vi "RT Main v1.05.vi"() -> ()   [LabVIEW 2017]
doc: "Changelog:\n\nv0.9:\n- Autocycle"
uses:
  Controls/Auto Delays.ctl
  support/Controls/General Para.ctl
  support/Controls/All Inputs.ctl
  support/Controls/Index Details.ctl
  support/Controls/Auto Stats.ctl
  Controls/Auto Times.ctl
  Global Variables/RT GV.vi
  support/Message Queue/Enqueue Message (Single).vi
  Global Variables/FPGA GV.vi
  <vilib>/Utility/error.llb/Error Cluster From Error Code.vi
  <vilib>/rvi/errors/niLvFpgaAdjustHostInterfaceError.vi
  Global Variables/Network Globals.vi
  <vilib>/FPGAPlugInAG/Dynamic/niLvFpga_Close_Dynamic.vi
  <vilib>/rvi/interface/nirviReadWriteControl/nirviReadWriteControl.xnode
  Controls/FPGA Ref.ctl
  <vilib>/rvi/interface/nirviCloseFPGA/nirviCloseFPGA.xnode
  support/Message Queue/Message Queue.lvlib
  NiFpgaLv.dll
  <vilib>/rvi/interface/Simulation/niFpgaSimulationCallBeginRW.vi
panel:
  in  "Auto Para":T1={"Agitator Delays"=[250, 350], "TF Delays"=[700, 800, 2], "Insertion Delays"=[100, 500], "Cutting Delays"=[300, 300, 100], "PF Delays"=[250, 30000], "Measur. Delays"=[500.0, 188.9, 1.0], "Reject Delays"=[500], "BF Delays"=[1000, 1000]}
  in  "Stop Button 4":bool
  out "error out":errorcluster
  out "Wrong Message":string
  in  "Stop Button":bool
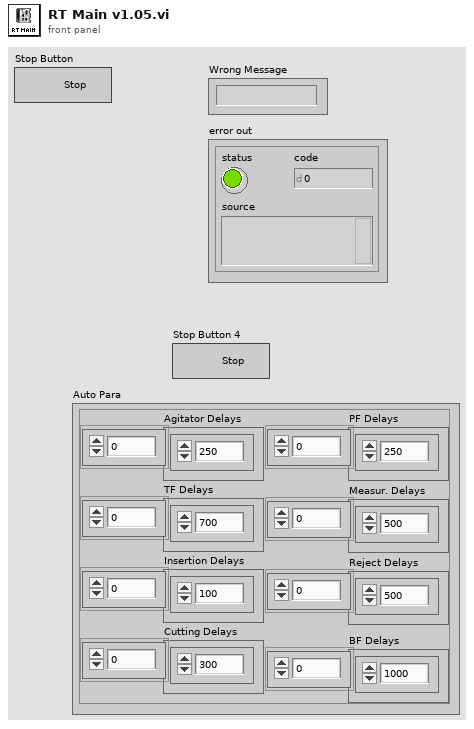
[diagram p1: front panel]
types:
  T1 = typedef "Auto Delays.ctl" = cluster{"Agitator Delays":u32[], "TF Delays":u32[], "Insertion Delays":u32[], "Cutting Delays":u32[], "PF Delays":u32[], "Measur. Delays":dbl[], "Reject Delays":u32[], "BF Delays":u32[]}
  T2 = typedef "FPGA Ref.ctl" = refnum<k20>
  T3 = cluster{"TL_Red":bool, "TL_Orange":bool, "TL_Green":bool, "TL_Buzzer":bool, "SOL_Index_Rotary_CW":bool, "SOL_Index_CNVR_Rotary_CCW":bool, "SOL_Index_CNVR_Stopper_Rear":bool, "SOL_Index_CNVR_Output _Separator _Rear":bool, "Bowl  Feeder_ ON":bool, "Pump_CNVR_Motor _ON":bool, "SOL_Gating_CYL_Rear":bool, "SOL_Tube_Feed_Agitatator":bool, "SOL_Tube_Feed_Gating_CYL":bool, "SOL_Insertion _CYL":bool, "SOL_Insertion_Clamp_CYL":bool, "SOL_Cutting_CYL":bool, "SOL_Cutting_Clamp_CYL":bool, "SOL_Insertion_Air_Nozzle":bool, "SOL_Measurement_CYL":bool, "SOL_Measure_Clamp_CYL":bool, "SOL_Rejection CYL_1":bool, "SOL_Rejection CYL_2":bool, "SOL_Rejection CYL_3":bool, "SOL_Rejection CYL_4":bool, "DO1.24":bool, "DO1.25":bool, "DO1.26":bool, "DO1.27":bool, "DO1.28":bool, "DO1.29":bool, "DO1.30":bool, "DO1.31":bool}
  T4 = typedef "General Para.ctl" = cluster{"Max. Cons.":dbl, "Offset 1":dbl, "Offset 2":dbl, "Offset 3":dbl, "Offset 4":dbl}
  T5 = typedef "All Inputs.ctl" = cluster{"DI 1":cluster{"Machine_ON":bool, "E_stop ":bool, "SW_Pressure":bool, "SW_Start ":bool, "SW_Reset":bool, "SW_Stop":bool, "SW_Door":bool, "RS_Index_Rotary_CW":bool, "RS_Index_Rotary_CCW":bool, "RS_Index_Stopper _Rear":bool, "RS_Index_Output_Separator_Rear":bool, "PES_Index_Pallet_Sensor":bool, "PES_Index_Output_Part Sensor":bool, "ICS_BF_Low_Level_1":bool, "ICS_BF_Low_Level_2":bool, "ICS_BF_Pump_CNVR_Full_1":bool, "ICS_BF_Pump_CNVR_Full_2":bool, "ICS_BF_Pump_CNVR_Full_3":bool, "ICS_BF_Pump_CNVR_Full_4":bool, "PES_PC_Pump Presence_1":bool, "PES_PC_Pump Presence_2":bool, "PES_PC_Pump Presence_3":bool, "PES_PC_Pump Presence_4":bool, "RS_PC_Gating_Front":bool, "PES_Pump_Interference":bool, "PES_TF_Low_Level":bool, "PES_Tube Presence_1":bool, "PES_Tube Presence_2":bool, "PES_Tube Presence_3":bool, "PES_Tube Presence_4":bool, "DI1.30":bool, "DI1.31":bool}, "DI 2":cluster{"RS_Agitatator_1_Rear ":bool, "RS_Agitatator_2_Rear ":bool, "RS_TF_Gating CYL_Rear":bool, "RS_Insertion_1_Rear":bool, "RS_Insertion_1_Front":bool, "RS_Insertion _2_Rear":bool, "RS_Insertion _2_Front":bool, "RS_Insertion _3_Rear":bool, "RS_Insertion _3_Front":bool, "RS_Insertion _4_Rear":bool, "RS_Insertion _4_Front":bool, "RS_Insertion_Clamp_Rear":bool, "RS_Cutting_Rear":bool, "RS_Cutting_Clamp _Rear":bool, "RS_Measurement_1_Rear":bool, "RS_Measurement_2_Rear":bool, "RS_Measurement_3_Rear":bool, "RS_Measurement_4_Rear":bool, "RS_Measure_Clamp_Rear":bool, "RS_Rejection_1_Rear":bool, "RS_Rejection_2_Rear":bool, "RS_Rejection_3_Rear":bool, "RS_Rejection_4_Rear":bool, "DI2.23":bool, "DI2.24":bool, "DI2.25":bool, "DI2.26":bool, "DI2.27":bool, "DI2.28":bool, "DI2.29":bool, "DI2.30":bool, "DI2.31":bool}, "IAS 1":dbl, "IAS 2":dbl, "IAS 3":dbl, "IAS 4":dbl, "DO 1":cluster{"TL_Red":bool, "TL_Orange":bool, "TL_Green":bool, "TL_Buzzer":bool, "SOL_Index_Rotary_CW":bool, "SOL_Index_CNVR_Rotary_CCW":bool, "SOL_Index_CNVR_Stopper_Rear":bool, "SOL_Index_CNVR_Output _Separator _Rear":bool, "Bowl  Feeder_ ON 1":bool, "Pump_CNVR_Motor _ON":bool, "SOL_PC_Gating_CYL_Rear":bool, "SOL_Tube_Feed_Agitatator":bool, "SOL_Tube_Feed_Gating_CYL":bool, "SOL_Insertion _CYL":bool, "SOL_Insertion_Clamp_CYL":bool, "SOL_Cutting_CYL":bool, "SOL_Cutting_Clamp_CYL":bool, "SOL_Insertion_Air_Nozzle":bool, "SOL_Measurement_CYL":bool, "DO1.19":bool, "SOL_Rejection CYL_1":bool, "SOL_Rejection CYL_2":bool, "SOL_Rejection CYL_3":bool, "SOL_Rejection CYL_4":bool, "Bowl  Feeder_ ON 2":bool, "SOL_BF_BlowerON":bool, "SOL_BF1_Track1":bool, "SOL_BF1_Track2":bool, "SOL_BF2_Track1":bool, "SOL_BF2_Track2":bool, "DO1.30":bool, "DO1.31":bool}}
  T6 = typedef "Index Details.ctl" = cluster{"Time (ms)":u32, "Waveform Graph":i16[]}
  T7 = cluster{T1, "Reject Pallets":cluster{"Reject 1":bool, "Reject 2":bool, "Reject 3":bool, "Reject 4":bool}}
  T8 = typedef "Auto Stats.ctl" = cluster{"Time-Stamp":timestamp, "Auto Times":T9, "Measurements":cluster{"1":dbl, "2":dbl, "3":dbl, "4":dbl}, "Outputs":cluster{"Good Parts":u32, "Reject Parts":u32}, "Cycle Time":dbl, "Remarks":string}
  T9 = typedef "Auto Times.ctl" = cluster{"Index Time":u32, "TF Time":u32, "Insertion Time":u32, "Cutting Time":u32, "PF Time":u32, "Meas. Time":u32, "Reject Time":u32}
  T10 = cluster{string, dbl, "cluster":cluster{"Auto Para":T1, "General Para":T4}}
  T11 = cluster{"TL_Red":bool, "TL_Orange":bool, "TL_Green":bool, "TL_Buzzer":bool, "SOL_Index_Rotary_CW":bool, "SOL_Index_CNVR_Rotary_CCW":bool, "SOL_Index_CNVR_Stopper_Rear":bool, "SOL_Index_CNVR_Output _Separator _Rear":bool, "Bowl Feeder_ ON1":bool, "Pump_CNVR_Motor _ON":bool, "SOL_PC_Gating_CYL_Rear":bool, "SOL_Tube_Feed_Agitatator":bool, "SOL_Tube_Feed_Gating_CYL":bool, "SOL_Insertion _CYL":bool, "SOL_Insertion_Clamp_CYL":bool, "SOL_Cutting_CYL":bool, "SOL_Cutting_Clamp_CYL":bool, "SOL_Insertion_Air_Nozzle":bool, "SOL_Measurement_CYL":bool, "DO1.19":bool, "SOL_Rejection CYL_1":bool, "SOL_Rejection CYL_2":bool, "SOL_Rejection CYL_3":bool, "SOL_Rejection CYL_4":bool, "Bowl Feeder_ON2":bool, "SOL_BF_BlowerON":bool, "SOL_BF1_Track1":bool, "SOL_BF1_Track2":bool, "SOL_BF2_Track1":bool, "SOL_BF2_Track2":bool, "DO1.30":bool, "DO1.31":bool}
  T12 = cluster{"Machine_ON":bool, "E_stop ":bool, "SW_Pressure":bool, "SW_Start ":bool, "SW_Reset":bool, "SW_Stop":bool, "SW_Door":bool, "RS_Index_Rotary_CW":bool, "RS_Index_Rotary_CCW":bool, "RS_Index_Stopper _Rear":bool, "RS_Index_Output_Separator_Rear":bool, "PES_Index_Pallet_Sensor":bool, "PES_Index_Output_Part Sensor":bool, "ICS_BF_Low_Level_1":bool, "ICS_BF_Low_Level_2":bool, "ICS_BF_Pump_CNVR_Full_1":bool, "ICS_BF_Pump_CNVR_Full_2":bool, "ICS_BF_Pump_CNVR_Full_3":bool, "ICS_BF_Pump_CNVR_Full_4":bool, "PES_PC_Pump Presence_1":bool, "PES_PC_Pump Presence_2":bool, "PES_PC_Pump Presence_3":bool, "PES_PC_Pump Presence_4":bool, "RS_PC_Gating_Front":bool, "PES_Pump_Interference":bool, "PES_TF_Low_Level":bool, "PES_Tube Presence_1":bool, "PES_Tube Presence_2":bool, "PES_Tube Presence_3":bool, "PES_Tube Presence_4":bool, "DI1.30":bool, "DI1.31":bool}
  T13 = cluster{"RS_Agitatator_1_Rear ":bool, "RS_Agitatator_2_Rear ":bool, "RS_TF_Gating CYL_Rear":bool, "RS_Insertion_1_Rear":bool, "RS_Insertion_1_Front":bool, "RS_Insertion _2_Rear":bool, "RS_Insertion _2_Front":bool, "RS_Insertion _3_Rear":bool, "RS_Insertion _3_Front":bool, "RS_Insertion _4_Rear":bool, "RS_Insertion _4_Front":bool, "RS_Insertion_Clamp_Rear":bool, "RS_Cutting_Rear":bool, "RS_Cutting_Clamp _Rear":bool, "RS_Measurement_1_Rear":bool, "RS_Measurement_2_Rear":bool, "RS_Measurement_3_Rear":bool, "RS_Measurement_4_Rear":bool, "DI2.18":bool, "RS_Rejection_1_Rear":bool, "RS_Rejection_2_Rear":bool, "RS_Rejection_3_Rear":bool, "RS_Rejection_4_Rear":bool, "DI2.23":bool, "DI2.24":bool, "DI2.25":bool, "DI2.26":bool, "DI2.27":bool, "DI2.28":bool, "DI2.29":bool, "DI2.30":bool, "DI2.31":bool}
  T14 = cluster{"Array":string[][], "Machine Status":string}
  T15 = cluster{"Measurements":cluster{"1":dbl, "2":dbl, "3":dbl, "4":dbl}, "Reject Pallets":cluster{"Reject 1":bool, "Reject 2":bool, "Reject 3":bool, "Reject 4":bool}}
  T16 = cluster{"Auto Times":T9, "Results":cluster{"Measurements":cluster{"1":dbl, "2":dbl, "3":dbl, "4":dbl}, "Reject Pallets":cluster{"Reject 1":bool, "Reject 2":bool, "Reject 3":bool, "Reject 4":bool}}, "OutputCount":u32, "error out":errorcluster}
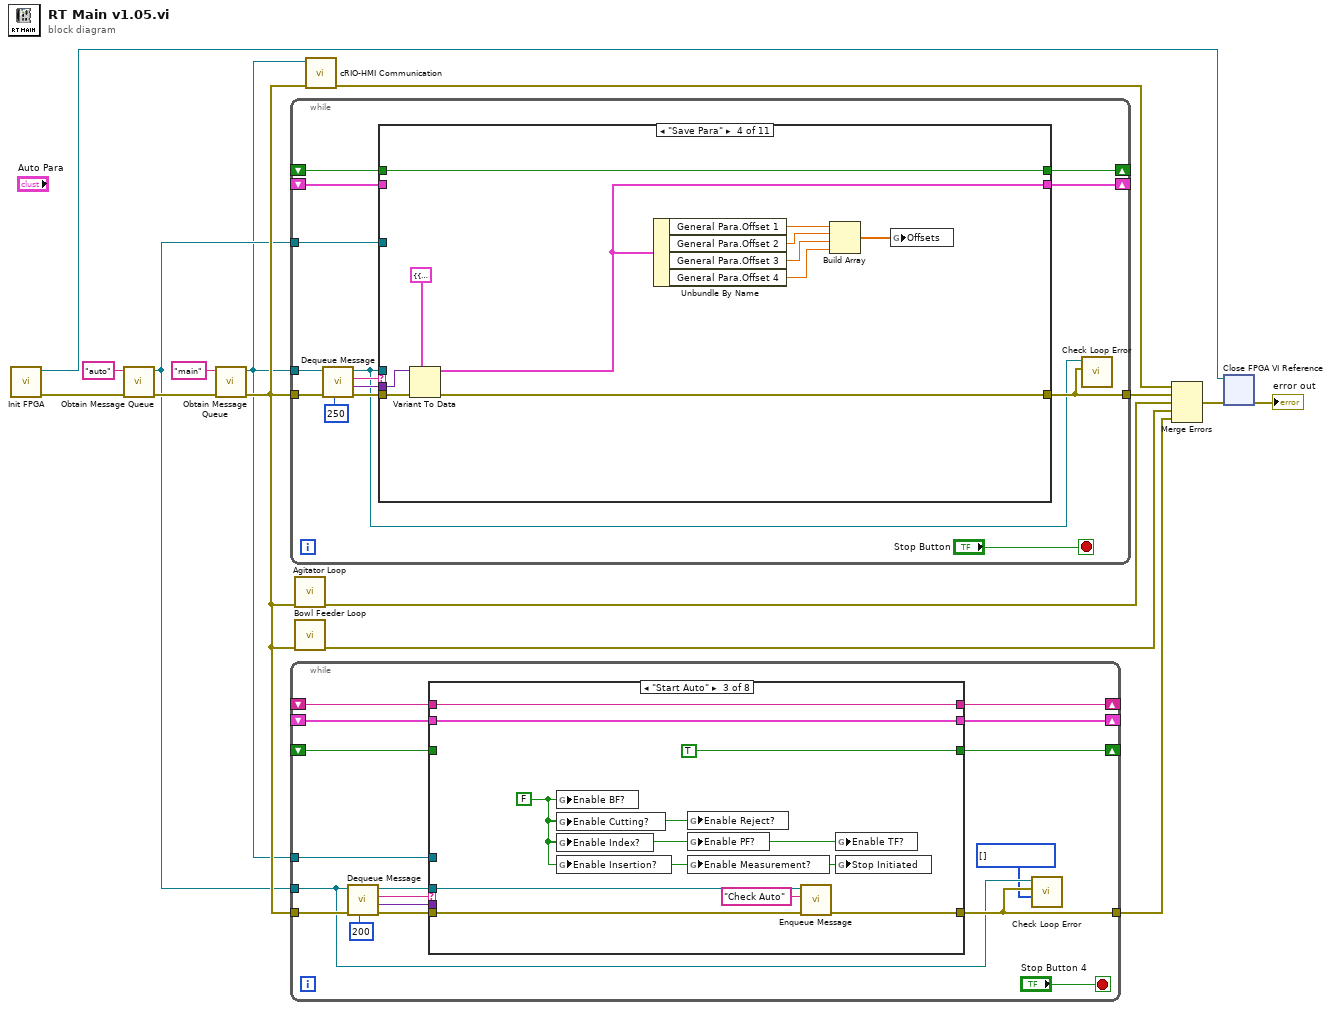
[diagram p0: block diagram]
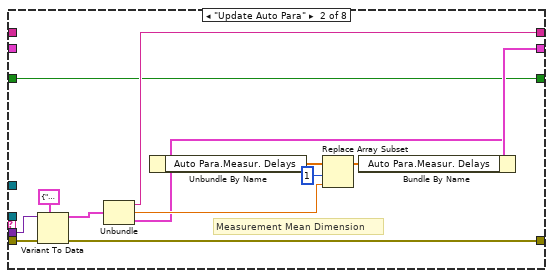
[diagram p3: hidden frame]
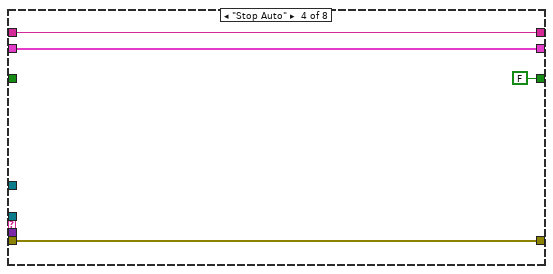
[diagram p4: hidden frame]
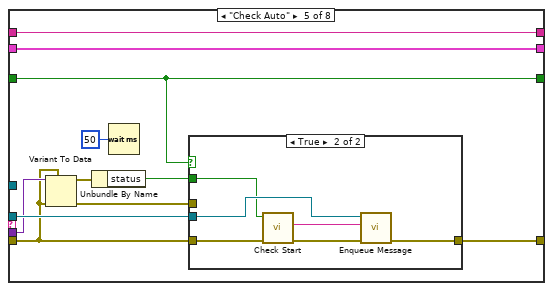
[diagram p5: hidden frame]
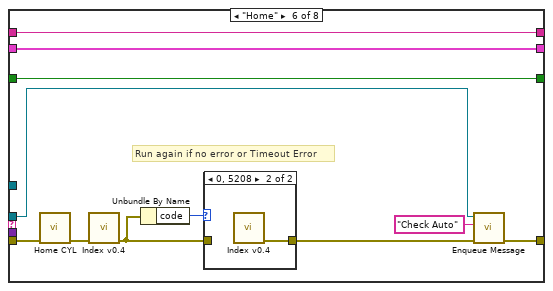
[diagram p7: hidden frame]
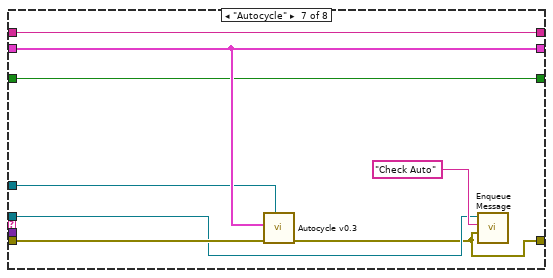
[diagram p9: hidden frame]
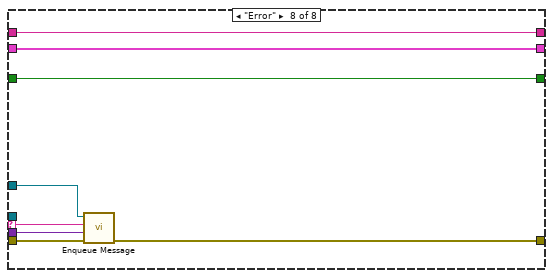
[diagram p10: hidden frame]
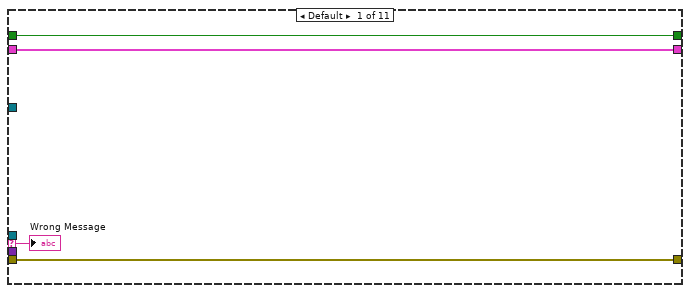
[diagram p11: hidden frame]
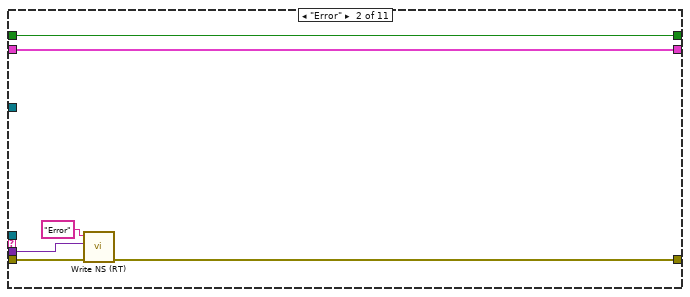
[diagram p12: hidden frame]
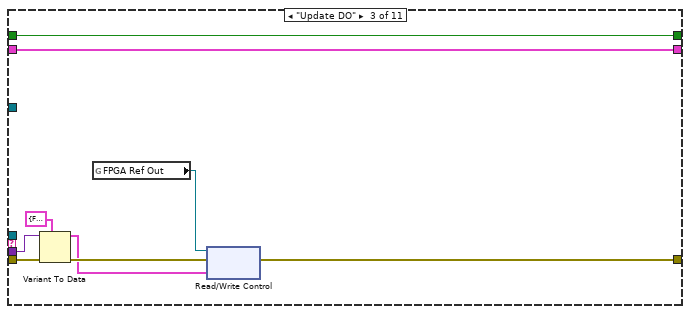
[diagram p13: hidden frame]
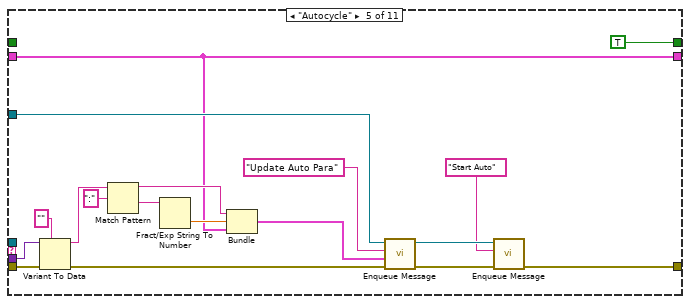
[diagram p14: hidden frame]
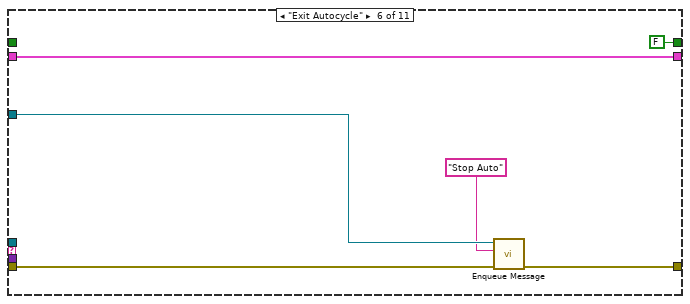
[diagram p15: hidden frame]
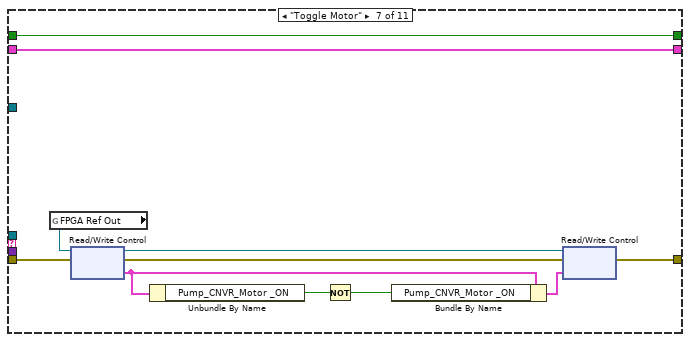
[diagram p16: hidden frame]
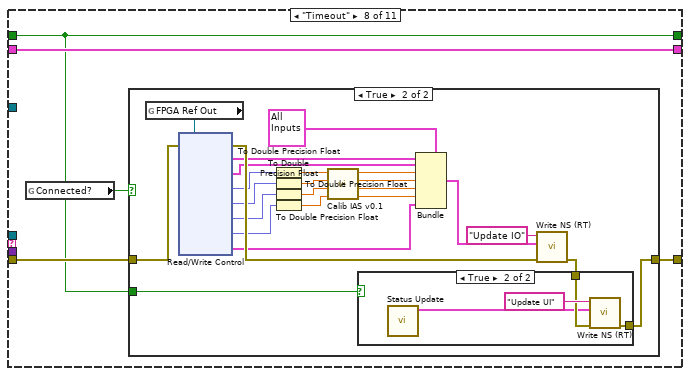
[diagram p17: hidden frame]
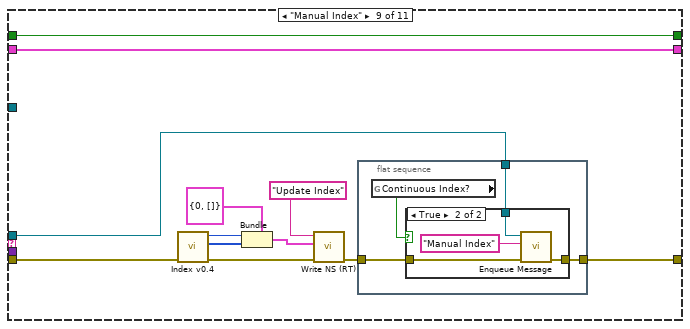
[diagram p20: hidden frame]
diagram:
  n1 = call "Init FPGA.vi"() -> ("error out"=w4:errorcluster, "FPGA Ref Out"=w9:T2)  [unwired: 10 in]
  n2 = call "Obtain Message Queue.vi"("error in (no error)"=w4, "name"="auto") -> ("error out"=w3:errorcluster, "Message Queue"=w2:refnum<queue>)  [unwired: 8 in]
  n3 = call "Obtain Message Queue.vi"("error in (no error)"=w3, "name"="main") -> ("error out"=w8:errorcluster, "Message Queue"=w1:refnum<queue>)  [unwired: 8 in]
  n4 = while {
    tunnel: w8 -> [w28]
    tunnel: w1 -> [w27]
    tunnel: [w23] -> w15
    tunnel: w2 -> [w20]
    shift-right: [w18] -> _
    shift-left: _ -> [w19]
    shift-right: [w16] -> _
    shift-left: _ -> [w17]
    stop <- "Stop Button" stop-if-true
    n5 = call "Dequeue Message.vi"("timeout"=250, "error in (no error)"=w28, "Message Queue"=w27) -> ("error out"=w26:errorcluster, "Message Data"=w24:variant, "Message"=w25:string, "dup Message Queue"=w22:refnum<queue>)  [unwired: 5 in]
    n6 = case shown="\"Save Para\"" w25 {
      selector: w25 -> [w33 _ _ _ _ _ _ _ _ _ _]
      tunnel: w26 -> [w32 w38 w48 w59 w77 w83 w93 w98 w141 w168 w178]
      tunnel: w22 -> [_ _ _ _ _ _ _ _ w133 _ _]
      tunnel: w24 -> [_ w36 w47 w58 w76 _ _ _ _ w167 w177]
      tunnel: [w32 w37 w43 w57 w63 w80 w91 w99 w134 w163 w174] -> w23
      tunnel: w20 -> [_ _ _ _ w69 w82 _ _ _ _ _]
      tunnel: w19 -> [w31 w39 w41 _ w66 w81 w85 w96 w131 w154 w173]
      tunnel: [w31 w39 w41 w54 w66 w81 w85 w96 w131 w154 w173] -> w18
      tunnel: w17 -> [w30 w34 w40 w56 _ _ w84 w95 w130 w151 w169]
      tunnel: [w30 w34 w40 w56 TRUE FALSE w84 w95 w130 w151 w169] -> w16
      frame Default {
        "Wrong Message" <- w33
      }
      frame "Error" {
        n7 = call "Write NS (RT).vi"("error in (no error)"=w38, "Message Data"=w36, "Message"="Error") -> ("error out"=w37:errorcluster)  [unwired: 8 in]
      }
      frame "Update DO" {
        n8 = Variant To Data(error in=w48, type=T3 {"TL_Red"=FALSE, "TL_Orange"=FALSE, "TL_Green"=FALSE, "TL_Buzzer"=FALSE, "SOL_Index_Rotary_CW"=FALSE, "SOL_Index_CNVR_Rotary_CCW"=FALSE, "SOL_Index_CNVR_Stopper_Rear"=FALSE, "SOL_Index_CNVR_Output _Separator _Rear"=FALSE, "Bowl  Feeder_ ON"=FALSE, "Pump_CNVR_Motor _ON"=FALSE, "SOL_Gating_CYL_Rear"=FALSE, "SOL_Tube_Feed_Agitatator"=FALSE, "SOL_Tube_Feed_Gating_CYL"=FALSE, "SOL_Insertion _CYL"=FALSE, "SOL_Insertion_Clamp_CYL"=FALSE, "SOL_Cutting_CYL"=FALSE, "SOL_Cutting_Clamp_CYL"=FALSE, "SOL_Insertion_Air_Nozzle"=FALSE, "SOL_Measurement_CYL"=FALSE, "SOL_Measure_Clamp_CYL"=FALSE, "SOL_Rejection CYL_1"=FALSE, "SOL_Rejection CYL_2"=FALSE, "SOL_Rejection CYL_3"=FALSE, "SOL_Rejection CYL_4"=FALSE, "DO1.24"=FALSE, "DO1.25"=FALSE, "DO1.26"=FALSE, "DO1.27"=FALSE, "DO1.28"=FALSE, "DO1.29"=FALSE, "DO1.30"=FALSE, "DO1.31"=FALSE} ("DO 1"), Variant=w47) -> (data=w42:T3, error out=w44:errorcluster)
        n9 = global read "FPGA GV.vi" "FPGA Ref Out"() -> (w45:T2)
        n10 = xnode "Read/Write Control"("FPGA VI Reference In"=w45, "error in"=w44, "DO 1"=w42) -> ("error out"=w43:errorcluster)  [unwired: 1 out]
      }
      frame "Save Para" {
        n11 = Variant To Data(error in=w59, type=cluster{"Auto Para":T1, "General Para":T4} {"Auto Para"={"Agitator Delays"=[], "TF Delays"=[], "Insertion Delays"=[], "Cutting Delays"=[], "PF Delays"=[], "Measur. Delays"=[], "Reject Delays"=[], "BF Delays"=[]}, "General Para"={"Max. Cons."=0.0, "Offset 1"=0.0, "Offset 2"=0.0, "Offset 3"=0.0, "Offset 4"=0.0}} ("cluster"), Variant=w58) -> (data=w54:cluster{"Auto Para":T1, "General Para":T4}, error out=w57:errorcluster)
        n12 = Unbundle By Name(w54) -> ("General Para.Offset 1"=w53:dbl, "General Para.Offset 2"=w52:dbl, "General Para.Offset 3"=w51:dbl, "General Para.Offset 4"=w50:dbl)
        n13 = Build Array(w53, w52, w51, w50) -> (w49:dbl[])
        n14 = global write "RT GV.vi" "Offsets"(w49) -> ()
      }
      frame "Autocycle" {
        n15 = Variant To Data(error in=w77, type="", Variant=w76) -> (data=w72:string, error out=w70:errorcluster)
        n16 = Match Pattern(string=w72, regular expression=":") -> (before substring=w68:string, after substring=w73:string)  [unwired: 1 in, 2 out]
        n17 = Fract/Exp String To Number(string=w73) -> (number=w67:dbl)  [unwired: 3 in, 1 out]
        n18 = Bundle(w68, w67, "cluster"=w66) -> (w65:T10)  [unwired: 1 in]
        n19 = call-poly "Enqueue Message.vi"("error in (no error)"=w70, "Message Data"=w65, "Message"="Update Auto Para", "Message Queue"=w69) -> ("error out"=w64:errorcluster, "dup Message Queue"=w62:refnum<queue>)  [unwired: 6 in]
        n20 = call-poly "Enqueue Message.vi"("error in (no error)"=w64, "Message"="Start Auto", "Message Queue"=w62) -> ("error out"=w63:errorcluster)  [unwired: 7 in, 1 out]
      }
      frame "Exit Autocycle" {
        n21 = call-poly "Enqueue Message.vi"("error in (no error)"=w83, "Message"="Stop Auto", "Message Queue"=w82) -> ("error out"=w80:errorcluster)  [unwired: 7 in, 1 out]
      }
      frame "Toggle Motor" {
        n22 = global read "FPGA GV.vi" "FPGA Ref Out"() -> (w94:T2)
        n23 = xnode "Read/Write Control"("FPGA VI Reference In"=w94, "error in"=w93) -> ("FPGA VI Reference Out"=w90:T2, "error out"=w92:errorcluster, "DO 1"=w88:T11)
        n24 = Unbundle By Name(w88) -> ("Pump_CNVR_Motor _ON"=w89:bool)
        n25 = Not(x=w89) -> (.not. x?=w86:bool)
        n26 = Bundle By Name(cluster=w88, "Pump_CNVR_Motor _ON"=w86) -> (w87:T11)
        n27 = xnode "Read/Write Control"("FPGA VI Reference In"=w90, "error in"=w92, "DO 1"=w87) -> ("error out"=w91:errorcluster)  [unwired: 1 out]
      }
      frame "Timeout" {
        n28 = global read "Network Globals.vi" "Connected?"() -> (w97:bool)
        n29 = case shown="True" w97 {
          tunnel: [w100 w103] -> w99
          tunnel: w98 -> [w100 w123]
          tunnel: w95 -> [_ w101]
          frame False {
          }
          frame True {
            n30 = global read "FPGA GV.vi" "FPGA Ref Out"() -> (w102:T2)
            n31 = xnode "Read/Write Control"("FPGA VI Reference In"=w102, "error in"=w123) -> ("error out"=w122:errorcluster, "DI 1"=w121:T12, "DI 2"=w120:T13, "AI0"=w119:fxp<+/-,27,6>, "AI1"=w118:fxp<+/-,27,6>, "AI2"=w117:fxp<+/-,27,6>, "AI3"=w116:fxp<+/-,27,6>, "DO 1"=w113:T11)  [unwired: 1 out]
            n32 = To Double Precision Float(number=w119) -> (double precision float=w106:dbl)
            n33 = To Double Precision Float(number=w118) -> (double precision float=w108:dbl)
            n34 = To Double Precision Float(number=w117) -> (double precision float=w110:dbl)
            n35 = To Double Precision Float(number=w116) -> (double precision float=w112:dbl)
            n36 = call "Calib IAS v0.1.vi"("x 4"=w112, "x 3"=w110, "x 2"=w108, "x"=w106) -> ("y 4"=w111:dbl, "y 3"=w109:dbl, "y 2"=w107:dbl, "y 1"=w105:dbl)  [unwired: 2 in, 2 out]
            n37 = Bundle(cluster=T5 {"DI 1"={"Machine_ON"=FALSE, "E_stop "=FALSE, "SW_Pressure"=FALSE, "SW_Start "=FALSE, "SW_Reset"=FALSE, "SW_Stop"=FALSE, "SW_Door"=FALSE, "RS_Index_Rotary_CW"=FALSE, "RS_Index_Rotary_CCW"=FALSE, "RS_Index_Stopper _Rear"=FALSE, "RS_Index_Output_Separator_Rear"=FALSE, "PES_Index_Pallet_Sensor"=FALSE, "PES_Index_Output_Part Sensor"=FALSE, "ICS_BF_Low_Level_1"=FALSE, "ICS_BF_Low_Level_2"=FALSE, "ICS_BF_Pump_CNVR_Full_1"=FALSE, "ICS_BF_Pump_CNVR_Full_2"=FALSE, "ICS_BF_Pump_CNVR_Full_3"=FALSE, "ICS_BF_Pump_CNVR_Full_4"=FALSE, "PES_PC_Pump Presence_1"=FALSE, "PES_PC_Pump Presence_2"=FALSE, "PES_PC_Pump Presence_3"=FALSE, "PES_PC_Pump Presence_4"=FALSE, "RS_PC_Gating_Front"=FALSE, "PES_Pump_Interference"=FALSE, "PES_TF_Low_Level"=FALSE, "PES_Tube Presence_1"=FALSE, "PES_Tube Presence_2"=FALSE, "PES_Tube Presence_3"=FALSE, "PES_Tube Presence_4"=FALSE, "DI1.30"=FALSE, "DI1.31"=FALSE}, "DI 2"={"RS_Agitatator_1_Rear "=FALSE, "RS_Agitatator_2_Rear "=FALSE, "RS_TF_Gating CYL_Rear"=FALSE, "RS_Insertion_1_Rear"=FALSE, "RS_Insertion_1_Front"=FALSE, "RS_Insertion _2_Rear"=FALSE, "RS_Insertion _2_Front"=FALSE, "RS_Insertion _3_Rear"=FALSE, "RS_Insertion _3_Front"=FALSE, "RS_Insertion _4_Rear"=FALSE, "RS_Insertion _4_Front"=FALSE, "RS_Insertion_Clamp_Rear"=FALSE, "RS_Cutting_Rear"=FALSE, "RS_Cutting_Clamp _Rear"=FALSE, "RS_Measurement_1_Rear"=FALSE, "RS_Measurement_2_Rear"=FALSE, "RS_Measurement_3_Rear"=FALSE, "RS_Measurement_4_Rear"=FALSE, "RS_Measure_Clamp_Rear"=FALSE, "RS_Rejection_1_Rear"=FALSE, "RS_Rejection_2_Rear"=FALSE, "RS_Rejection_3_Rear"=FALSE, "RS_Rejection_4_Rear"=FALSE, "DI2.23"=FALSE, "DI2.24"=FALSE, "DI2.25"=FALSE, "DI2.26"=FALSE, "DI2.27"=FALSE, "DI2.28"=FALSE, "DI2.29"=FALSE, "DI2.30"=FALSE, "DI2.31"=FALSE}, "IAS 1"=0.0, "IAS 2"=0.0, "IAS 3"=0.0, "IAS 4"=0.0, "DO 1"={"TL_Red"=FALSE, "TL_Orange"=FALSE, "TL_Green"=FALSE, "TL_Buzzer"=FALSE, "SOL_Index_Rotary_CW"=FALSE, "SOL_Index_CNVR_Rotary_CCW"=FALSE, "SOL_Index_CNVR_Stopper_Rear"=FALSE, "SOL_Index_CNVR_Output _Separator _Rear"=FALSE, "Bowl  Feeder_ ON 1"=FALSE, "Pump_CNVR_Motor _ON"=FALSE, "SOL_PC_Gating_CYL_Rear"=FALSE, "SOL_Tube_Feed_Agitatator"=FALSE, "SOL_Tube_Feed_Gating_CYL"=FALSE, "SOL_Insertion _CYL"=FALSE, "SOL_Insertion_Clamp_CYL"=FALSE, "SOL_Cutting_CYL"=FALSE, "SOL_Cutting_Clamp_CYL"=FALSE, "SOL_Insertion_Air_Nozzle"=FALSE, "SOL_Measurement_CYL"=FALSE, "DO1.19"=FALSE, "SOL_Rejection CYL_1"=FALSE, "SOL_Rejection CYL_2"=FALSE, "SOL_Rejection CYL_3"=FALSE, "SOL_Rejection CYL_4"=FALSE, "Bowl  Feeder_ ON 2"=FALSE, "SOL_BF_BlowerON"=FALSE, "SOL_BF1_Track1"=FALSE, "SOL_BF1_Track2"=FALSE, "SOL_BF2_Track1"=FALSE, "SOL_BF2_Track2"=FALSE, "DO1.30"=FALSE, "DO1.31"=FALSE}}, "DI 1"=w121, "DI 2"=w120, "IAS 1"=w105, "IAS 2"=w107, "IAS 3"=w109, "IAS 4"=w111, "DO 1"=w113) -> (w115:T5)
            n38 = call "Write NS (RT).vi"("error in (no error)"=w122, "Message Data"=w115, "Message"="Update IO") -> ("error out"=w104:errorcluster)  [unwired: 8 in]
            n39 = case shown="True" w101 {
              tunnel: w104 -> [w125 w128]
              tunnel: [w125 w127] -> w103
              frame False {
              }
              frame True {
                n40 = call "Status Update.vi"() -> ("Status Cluster"=w126:T14)  [unwired: 11 in]
                n41 = call "Write NS (RT).vi"("error in (no error)"=w128, "Message Data"=w126, "Message"="Update UI") -> ("error out"=w127:errorcluster)  [unwired: 8 in]
              }
            }
          }
        }
      }
      frame "Manual Index" {
        n42 = call "Index v0.4.vi"("error in (no error)"=w141) -> ("error out"=w139:errorcluster, "Waveform Graph"=w137:i16[], "Index Time"=w138:u32)  [unwired: 7 in, 1 out]
        n43 = Bundle(cluster=T6 {"Time (ms)"=0, "Waveform Graph"=[]}, "Time (ms)"=w138, "Waveform Graph"=w137) -> (w136:T6)
        n44 = call "Write NS (RT).vi"("error in (no error)"=w139, "Message Data"=w136, "Message"="Update Index") -> ("error out"=w135:errorcluster)  [unwired: 8 in]
        n45 = flat-sequence {
          tunnel: w135 -> [w145]
          tunnel: [w144] -> w134
          tunnel: w133 -> [w142]
          frame #0 {
            n46 = global read "RT GV.vi" "Continuous Index?"() -> (w143:bool)
            n47 = case shown="True" w143 {
              tunnel: w145 -> [w146 w150]
              tunnel: [w146 w149] -> w144
              tunnel: w142 -> [_ w147]
              frame False {
              }
              frame True {
                n48 = call-poly "Enqueue Message.vi"("error in (no error)"=w150, "Message"="Manual Index", "Message Queue"=w147) -> ("error out"=w149:errorcluster)  [unwired: 7 in, 1 out]
              }
            }
          }
        }
      }
      frame "Manual Run" {
        n49 = Variant To Data(error in=w168, type=T7 {{"Agitator Delays"=[1000], "TF Delays"=[1000], "Insertion Delays"=[1000], "Cutting Delays"=[1000], "PF Delays"=[1000], "Measur. Delays"=[1000.0], "Reject Delays"=[1000], "BF Delays"=[1000]}, "Reject Pallets"={"Reject 1"=FALSE, "Reject 2"=FALSE, "Reject 3"=FALSE, "Reject 4"=FALSE}}, Variant=w167) -> (data=w159:T7, error out=w166:errorcluster)
        n50 = Unbundle(w159) -> (w156:T1)  [unwired: 1 out]
        n51 = Unbundle By Name(w156) -> ("Agitator Delays"=w153:u32[], "BF Delays"=w152:u32[])
        n52 = call "Manual.vi"("error in"=w166, "Auto Delays"=w156) -> ("error out"=w158:errorcluster, "OutputCount"=w157:u32, "Results"=w155:T15, "Auto Times"=w162:T9)  [unwired: 6 in]
        n53 = global write "RT GV.vi" "Agitator Delays"(w153) -> ()
        n54 = global write "RT GV.vi" "BF Delays"(w152) -> ()
        n55 = Bundle("Auto Times"=w162, "Results"=w155, "OutputCount"=w157, "error out"=w158) -> (w161:T16)  [unwired: 1 in]
        n56 = call "Write NS (RT).vi"("Message Data"=w161, "Message"="Manual Status") -> ("error out"=w164:errorcluster)  [unwired: 9 in]
        n57 = Merge Errors(w164) -> (w163:errorcluster)
      }
      frame "Log Cycle" {
        n58 = Variant To Data(error in=w178, type=T8 {"Time-Stamp"=timestamp(0 s since 1904-01-01), "Auto Times"={"Index Time"=0, "TF Time"=0, "Insertion Time"=0, "Cutting Time"=0, "PF Time"=0, "Meas. Time"=0, "Reject Time"=0}, "Measurements"={"1"=0.0, "2"=0.0, "3"=0.0, "4"=0.0}, "Outputs"={"Good Parts"=0, "Reject Parts"=0}, "Cycle Time"=0.0, "Remarks"=""} ("Auto Stats"), Variant=w177) -> (data=w170:T8, error out=w171:errorcluster)
        n59 = call "Write NS (RT).vi"("error in (no error)"=w171, "Message Data"=w170, "Message"="Autocycle Log") -> ("error out"=w175:errorcluster)  [unwired: 8 in]
        n60 = Merge Errors(w175) -> (w174:errorcluster)
      }
    }
    n61 = call "Check Loop Error.vi"("error to process"=w23, "Message Queue"=w22) -> ()  [unwired: 8 in, 2 out]
  }
  n62 = while {
    tunnel: w8 -> [w193]
    tunnel: [w191] -> w7
    tunnel: w2 -> [w183]
    shift-right: [w187] -> _
    shift-left: _ -> [w186]
    shift-right: [w185] -> _
    shift-left: _ -> [w184]
    shift-right: [w182] -> _
    shift-left: _ -> [w181]
    tunnel: w1 -> [w180]
    stop <- "Stop Button 4" stop-if-true
    n63 = call "Dequeue Message.vi"("timeout"=200, "error in (no error)"=w193, "Message Queue"=w183) -> ("error out"=w192:errorcluster, "Message Data"=w188:variant, "Message"=w189:string, "dup Message Queue"=w190:refnum<queue>)  [unwired: 5 in]
    n64 = case shown="\"Start Auto\"" w189 {
      selector: w189 -> [_ _ _ _ _ _ _ w268]
      tunnel: w192 -> [w199 w212 w217 w222 w227 w250 w263 w266]
      tunnel: [w199 w211 w216 w222 w233 w245 w256 w265] -> w191
      tunnel: w190 -> [_ _ w215 _ w232 w243 w257 _]
      tunnel: w188 -> [_ w210 _ _ w229 _ _ w267]
      tunnel: [w198 w208 w220 w224 w235 w253 w262 w271] -> w187
      tunnel: w186 -> [w198 _ w220 w224 w235 w253 w262 w271]
      tunnel: [w197 w203 w219 w223 w234 w252 w261 w270] -> w185
      tunnel: w184 -> [w197 _ w219 w223 w234 w252 w261 w270]
      tunnel: [w196 w202 TRUE FALSE w231 w251 w259 w269] -> w182
      tunnel: w181 -> [w196 w202 _ _ w231 w251 w259 w269]
      tunnel: w180 -> [_ _ _ _ _ _ w260 w264]
      frame Default {
      }
      frame "Update Auto Para" {
        # "Measurement Mean Dimension"
        n65 = Variant To Data(error in=w212, type=T10 {"", 0.0, "cluster"={"Auto Para"={"Agitator Delays"=[], "TF Delays"=[], "Insertion Delays"=[], "Cutting Delays"=[], "PF Delays"=[], "Measur. Delays"=[], "Reject Delays"=[], "BF Delays"=[]}, "General Para"={"Max. Cons."=0.0, "Offset 1"=0.0, "Offset 2"=0.0, "Offset 3"=0.0, "Offset 4"=0.0}}} ("cluster"), Variant=w210) -> (data=w209:T10, error out=w211:errorcluster)
        n66 = Unbundle(w209) -> (w208:string, w205:dbl, "cluster"=w201:cluster{"Auto Para":T1, "General Para":T4})
        n67 = Unbundle By Name(w201) -> ("Auto Para.Measur. Delays"=w207:dbl[])
        n68 = Replace Array Subset(array=w207, new element=w205, index=1) -> (w204:dbl[])
        n69 = Bundle By Name(cluster=w201, "Auto Para.Measur. Delays"=w204) -> (w203:cluster{"Auto Para":T1, "General Para":T4})
      }
      frame "Start Auto" {
        w213 = FALSE ("Enable BF?")
        n70 = global write "RT GV.vi" "Enable BF?"(w213) -> ()
        n71 = global write "RT GV.vi" "Enable Cutting?"(w213) -> ()
        n72 = global write "RT GV.vi" "Enable Index?"(w213) -> ()
        n73 = global write "RT GV.vi" "Enable Insertion?"(w213) -> ()
        n74 = global write "RT GV.vi" "Enable Reject?"(w213) -> ()
        n75 = global write "RT GV.vi" "Enable PF?"(w213) -> ()
        n76 = global write "RT GV.vi" "Enable Measurement?"(w213) -> ()
        n77 = call-poly "Enqueue Message.vi"("error in (no error)"=w217, "Message"="Check Auto", "Message Queue"=w215) -> ("error out"=w216:errorcluster)  [unwired: 7 in, 1 out]
        n78 = global write "RT GV.vi" "Enable TF?"(w213) -> ()
        n79 = global write "RT GV.vi" "Stop Initiated"(w213) -> ()
      }
      frame "Stop Auto" {
      }
      frame "Check Auto" {
        n80 = Variant To Data(error in=w227, type=w227, Variant=w229) -> (data=w226:errorcluster, error out=w228:errorcluster)
        n81 = Unbundle By Name(w226) -> ("status"=w225:bool)
        n82 = Wait (ms)(milliseconds to wait=u32 50) -> ()  [unwired: 1 out]
        n83 = case shown="True" w231 {
          tunnel: [w236 w242] -> w233
          tunnel: w232 -> [_ w238]
          tunnel: w227 -> [w236 w241]
          tunnel: w228 -> [_ _]
          tunnel: w225 -> [_ w237]
          frame False {
          }
          frame True {
            n84 = call "Check Start.vi"("error in"=w241, "Error Stop?"=w237) -> ("error out"=w240:errorcluster, "Message"=w239:string)  [unwired: 8 in]
            n85 = call-poly "Enqueue Message.vi"("error in (no error)"=w240, "Message"=w239, "Message Queue"=w238) -> ("error out"=w242:errorcluster)  [unwired: 7 in, 1 out]
          }
        }
      }
      frame "Home" {
        # "Run again if no error or Timeout Error"
        n86 = call "Home CYL.vi"("error in"=w250) -> ("error out"=w249:errorcluster)  [unwired: 10 in]
        n87 = call "Index v0.4.vi"("error in (no error)"=w249) -> ("error out"=w247:errorcluster)  [unwired: 7 in, 3 out]
        n88 = Unbundle By Name(w247) -> ("code"=w248:i32)
        n89 = case shown="0, 5208" w248 {
          tunnel: [w254 w255] -> w244
          tunnel: w247 -> [w254 _]
          frame Default {
          }
          frame 0, 5208 {
            n90 = call "Index v0.4.vi"() -> ("error out"=w255:errorcluster)  [unwired: 8 in, 3 out]
          }
        }
        n91 = call-poly "Enqueue Message.vi"("error in (no error)"=w244, "Message"="Check Auto", "Message Queue"=w243) -> ("error out"=w245:errorcluster)  [unwired: 7 in, 1 out]
      }
      frame "Autocycle" {
        n92 = call "Autocycle v0.3.vi"("Message Queue"=w260, "error in"=w263, "All Para"=w261) -> ("error out"=w256:errorcluster)  [unwired: 8 in]
        n93 = call-poly "Enqueue Message.vi"("Message Data"=w256, "Message"="Check Auto", "Message Queue"=w257) -> ()  [unwired: 7 in, 2 out]
      }
      frame "Error" {
        n94 = call-poly "Enqueue Message.vi"("error in (no error)"=w266, "Message Data"=w267, "Message"=w268, "Message Queue"=w264) -> ("error out"=w265:errorcluster)  [unwired: 6 in, 1 out]
      }
    }
    n95 = call "Check Loop Error.vi"("Ignore Errors"=i32[] [], "error to process"=w191, "Message Queue"=w183) -> ()  [unwired: 7 in, 2 out]
  }
  n96 = call "Agitator Loop.vi"("error in (no error)"=w8) -> ("error out"=w11:errorcluster)  [unwired: 10 in]
  n97 = call "Bowl Feeder Loop.vi"("error in (no error)"=w8) -> ("error out"=w10:errorcluster)  [unwired: 10 in]
  n98 = call "cRIO-HMI Communication.vi"("error in (no error)"=w8, "Message Queue"=w1) -> ("error out"=w14:errorcluster)  [unwired: 9 in]
  n99 = Merge Errors(w14, w15, w11, w10, w7) -> (w13:errorcluster)
  n100 = xnode ("Close FPGA VI Reference")("FPGA VI Reference In"=w9, "error in"=w13) -> ("error out"=→"error out":errorcluster)
